vi "Loop.vi"(11 "eeeee in":refnum<class "eeeee.lvclass">) -> (3 "eeeee out":refnum<class "eeeee.lvclass">)   [LabVIEW 2021, in "jettl Tools.lvlib" / "eeeee.lvlib" / "eeeee.lvclass"]
uses:
  eeeee.lvclass
  C:/git/jettl/src/jettl/jettl/jettl.lvclass
  eeeee.lvclass/eeeee.ctl
  jettl/Event/Event.lvclass
  jettl/Msg Strategy/Msg Strategy.lvclass
  C:/git/jettl/src/jettl Msg Merge Error/jettl Msg Merge Error/jettl Msg Merge Error.lvclass
  C:/git/jettl/src/jettl/Event/Event.lvclass
  C:/git/jettl/src/jettl Msg Override Error/jettl Msg Override Error/jettl Msg Override Error.lvclass
  C:/git/jettl/src/jettl Msg Setup/jettl Msg Setup/jettl Msg Setup.lvclass
  C:/git/jettl/src/jettl Msg Teardown/jettl Msg Teardown/jettl Msg Teardown.lvclass
  C:/git/jettl/src/jettl Tools/eeeee/eeeee/eeeee.lvclass
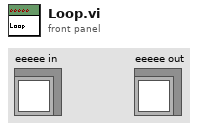
[diagram p1: front panel]
types:
  T1 = cluster{"Registration":refnum<event-registration>}
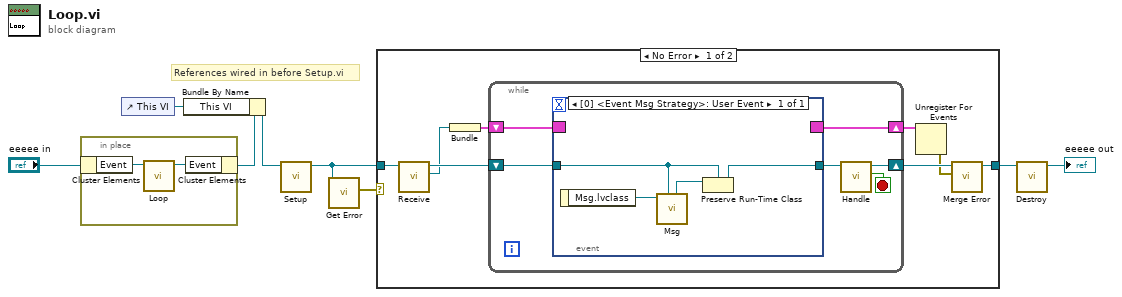
[diagram p0: block diagram]
diagram:
  # "References wired in before Setup.vi"
  n1 = in-place {
    n2 = in-place-cluster #1("eeeee in") -> ("Event"=w10:refnum<class "Event.lvclass">)
    n3 = call-dynamic "Loop.vi"("Event in"=w10) -> ("Event out"=w9:refnum<class "Event.lvclass">)  [unwired: 10 in]
    n4 = in-place-cluster #1("Event"=w9) -> (w7:refnum<class "eeeee.lvclass">)
  }
  n5 = control-ref of="This VI"() -> (w6:refnum<vi>)
  n6 = Bundle By Name(cluster=w7, "This VI"=w6) -> (w5:refnum<class "eeeee.lvclass">)
  n7 = call-dynamic "Setup.vi"("eeeee in"=w5) -> ("eeeee out"=w4:refnum<class "eeeee.lvclass">)  [unwired: 10 in]
  n8 = call-dynamic "Get Error.vi"("eeeee in"=w4) -> ("Error"=w3:errorcluster)  [unwired: 10 in]
  n9 = case shown="No Error" w3 {
    tunnel: w4 -> [w18 w29]
    tunnel: [w12 w29] -> w2
    frame No Error {
      n10 = call-dynamic "Receive.vi"("eeeee in"=w18) -> ("Registration"=w15:refnum<event-registration>, "eeeee out"=w17:refnum<class "eeeee.lvclass">)  [unwired: 9 in]
      n11 = Bundle("Registration"=w15) -> (w16:T1)  [unwired: 1 in]
      n12 = while {
        shift-right: [w19] -> w13
        shift-left: w17 -> [w23]
        shift-right: [w22] -> w14
        shift-left: w16 -> [w24]
        stop <- w21 stop-if-true
        n13 = event shown="[0] <Event Msg Strategy>: User Event" {
          selector: w24 -> [_]
          dyn-events: [_] -> w22
          timeout: _ -> [_]
          tunnel: [w25] -> w20
          tunnel: w23 -> [w26]
          event User Event {
            n14 = event-data() -> ("Msg.lvclass"=w28:refnum<class "Msg Strategy.lvclass">)  [unwired: 1 in]
            n15 = call-dynamic "Msg.vi"("jettl in"=w26, "Msg Strategy in"=w28) -> ("jettl out"=w27:refnum<class "jettl.lvclass">)  [unwired: 9 in]
            n16 = Preserve Run-Time Class(object in=w27, 2:w26) -> (object out=w25:refnum<class "eeeee.lvclass">)  [unwired: 1 in, 1 out]
          }
        }
        n17 = call-dynamic "Handle.vi"("eeeee in"=w20) -> ("Destroy?"=w21:bool, "eeeee out"=w19:refnum<class "eeeee.lvclass">)  [unwired: 9 in]
      }
      n18 = Unregister For Events(event registration refnum=w14) -> (error out=w11:errorcluster)  [unwired: 1 in]
      n19 = call-dynamic "Merge Error.vi"("Error"=w11, "eeeee in"=w13) -> ("eeeee out"=w12:refnum<class "eeeee.lvclass">)  [unwired: 9 in]
    }
    frame Error {
    }
  }
  n20 = call-dynamic "Destroy.vi"("eeeee in"=w2) -> ("eeeee out"=→"eeeee out":refnum<class "eeeee.lvclass">)  [unwired: 10 in]
